vi "Can Grabber.vi"(10 "Grabber State":dbl) -> ()   [LabVIEW 2014]
uses:
  Begin/Global Variables.vi
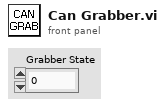
[diagram p1: front panel]
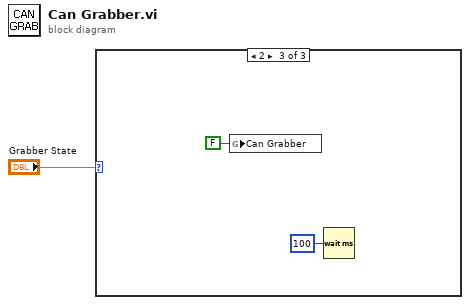
[diagram p0: block diagram]
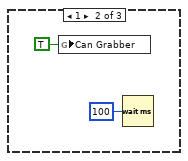
[diagram p3: hidden frame]
diagram:
  n1 = case shown="2" "Grabber State" {
    frame 0, Default {
    }
    frame 1 {
      n2 = global write "Global Variables.vi" "Can Grabber"(TRUE ("Can Grabber")) -> ()
      n3 = Wait (ms)(milliseconds to wait=u32 100) -> ()  [unwired: 1 out]
    }
    frame 2 {
      n4 = global write "Global Variables.vi" "Can Grabber"(FALSE ("Can Grabber")) -> ()
      n5 = Wait (ms)(milliseconds to wait=u32 100) -> ()  [unwired: 1 out]
    }
  }
